vi "WritePropertiesToVariant.vi"(8 "error in (no error)":errorcluster, 10 "Key Value Properties":T1[](array[typedef]), 11 "Variant Properties":variant) -> (0 "error out":errorcluster, 3 "Variant Properties Out":variant)   [LabVIEW 2017, in "AnalysisHelper.lvlib"]
uses:
  <vilib>/addons/InsightCM/Utilities/Analysis/Shared/AnalysisHelper.lvlib
  <vilib>/addons/InsightCM/MessageBus/Base/controls/KeyValuePair.ctl
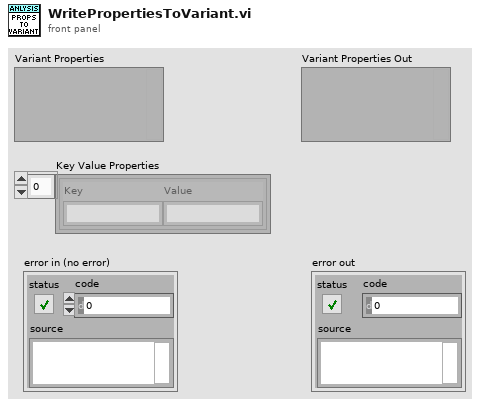
[diagram p1: front panel]
types:
  T1 = typedef "KeyValuePair.ctl" = cluster{"Key":string, "Value":string}
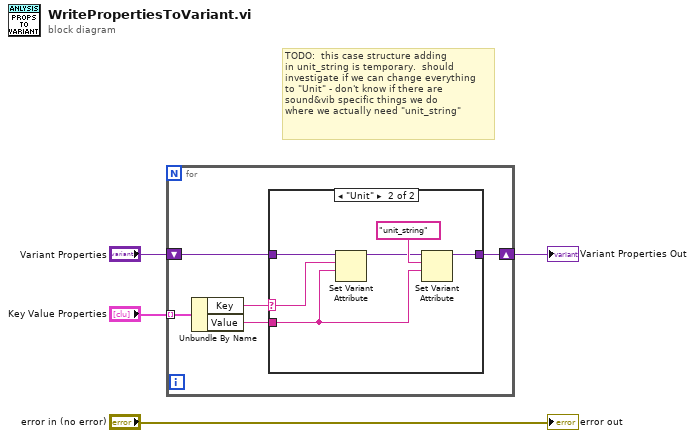
[diagram p0: block diagram]
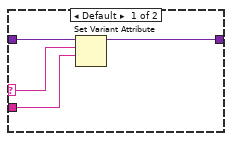
[diagram p2: hidden frame]
diagram:
  # "TODO:  this case structure adding\nin unit_string is temporary.  should\ninvestigate if we can change everything\nto \"Unit\" - don't know if there are\nsound&vib specific things we do\nwhere we actually need \"unit_string\""
  n1 = for {
    shift-right: [w5] -> w3
    shift-left: "Variant Properties" -> [w9]
    tunnel: "Key Value Properties" -> [w8] mode=indexing
    n2 = Unbundle By Name(w8) -> ("Key"=w6:string, "Value"=w7:string)
    n3 = case shown="\"Unit\"" w6 {
      selector: w6 -> [w10 w18]
      tunnel: w9 -> [w13 w19]
      tunnel: [w12 w15] -> w5
      tunnel: w7 -> [w11 w14]
      frame Default {
        n4 = Set Variant Attribute(Variant=w13, name=w10, value=w11) -> (Variant out=w12:variant)  [unwired: 1 in, 2 out]
      }
      frame "Unit" {
        n5 = Set Variant Attribute(Variant=w19, name=w18, value=w14) -> (Variant out=w16:variant)  [unwired: 1 in, 2 out]
        n6 = Set Variant Attribute(Variant=w16, name="unit_string", value=w14) -> (Variant out=w15:variant)  [unwired: 1 in, 2 out]
      }
    }
  }
  "Variant Properties Out" <- w3
  "error out" <- "error in (no error)"
